vi "数据查询_仪器数据.vi"() -> ()   [LabVIEW 2016]
uses:
  <vilib>/Utility/miscctls.llb/LVRowAndColumnUnsignedTypeDef.ctl
  <vilib>/Utility/miscctls.llb/LVPointTypeDef.ctl
panel:
  in  "工作模式":string(combo)="全部数据"
  in  "查询":bool
  in  "结束日期":string="2020/01/01"
  in  "起始日期":string="2010/01/01"
  in  "组合框":string(combo)
  out "数据表":string[][](table)
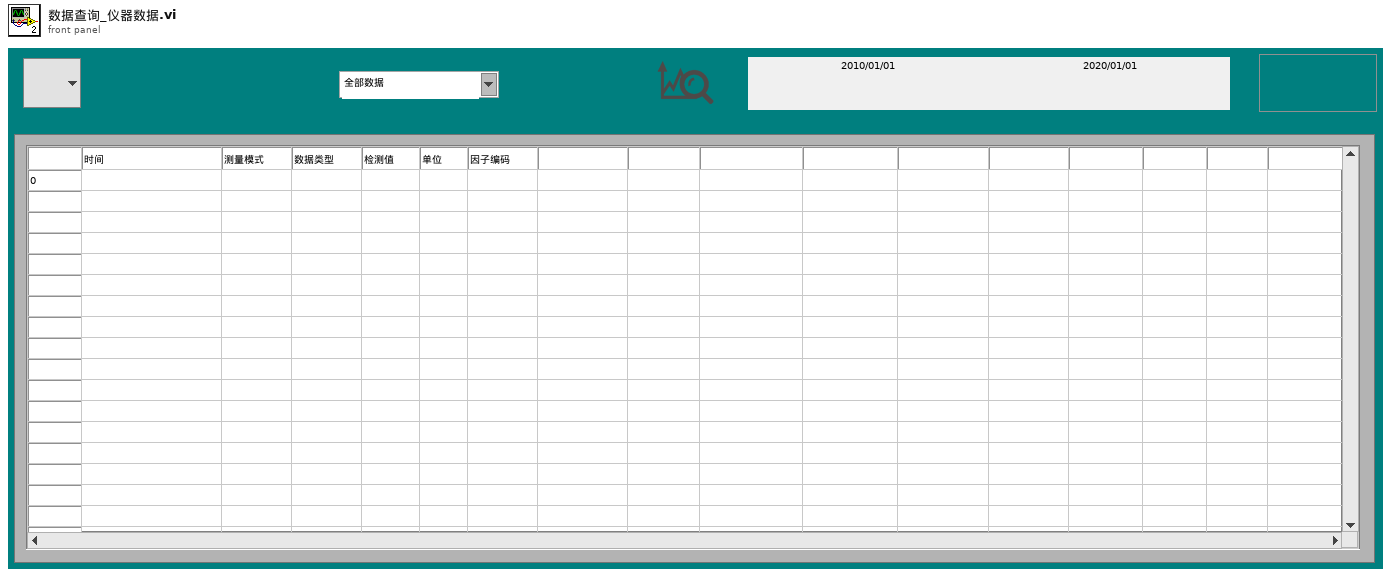
[diagram p1: front panel]
types:
  T1 = typedef "LVRowAndColumnUnsignedTypeDef.ctl" = cluster{"Row":u32, "Column":u32}
  T2 = typedef "LVPointTypeDef.ctl" = cluster{"Horizontal":i16, "Vertical":i16}
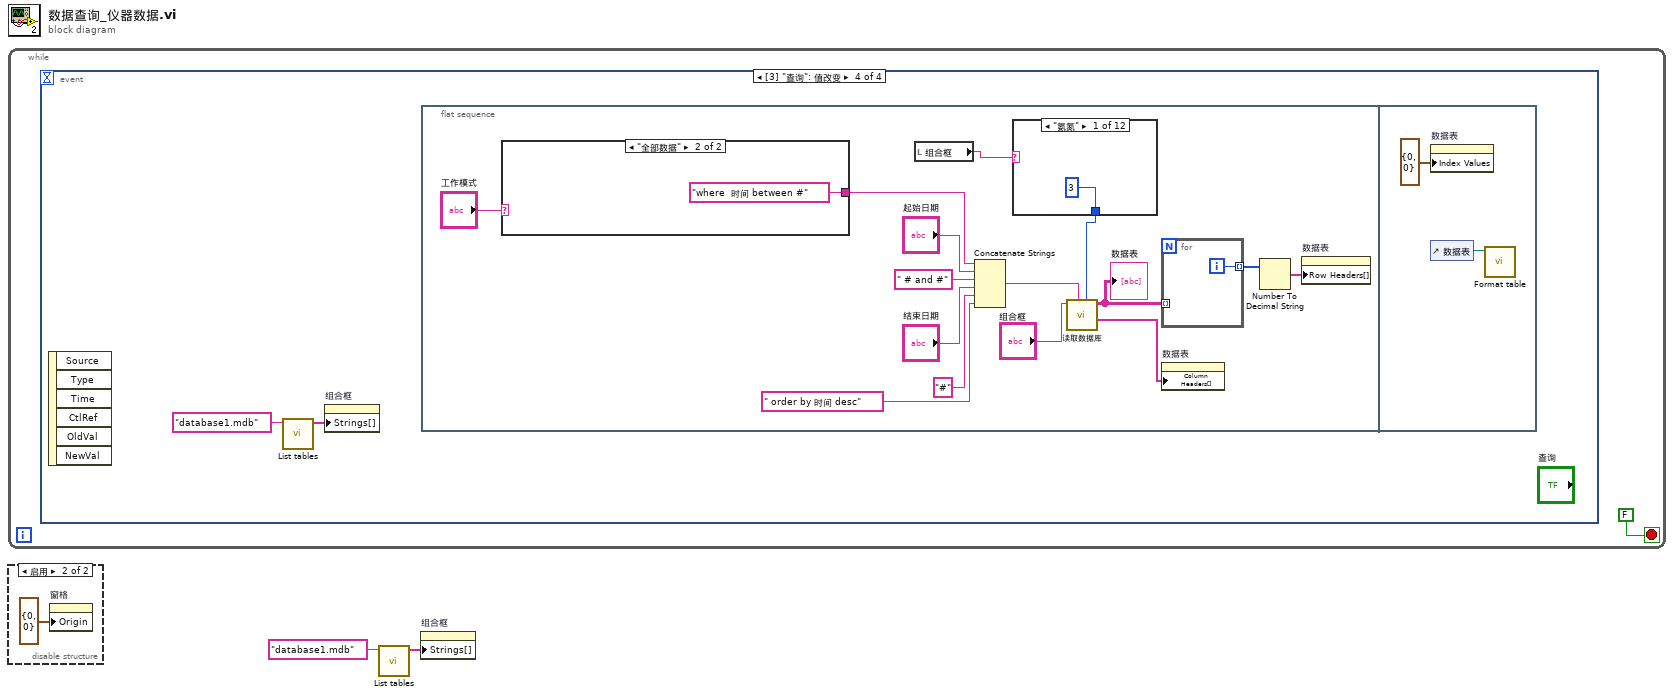
[diagram p0: block diagram]
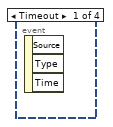
[diagram p2: hidden frame]
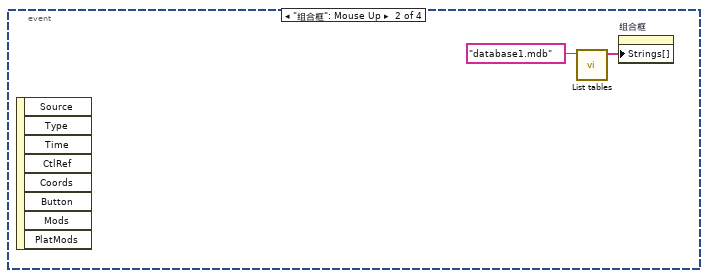
[diagram p3: hidden frame]
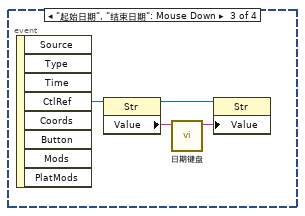
[diagram p4: hidden frame]
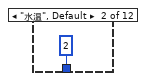
[diagram p5: hidden frame]
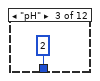
[diagram p6: hidden frame]
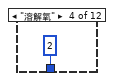
[diagram p7: hidden frame]
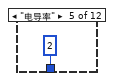
[diagram p8: hidden frame]
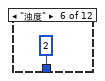
[diagram p9: hidden frame]
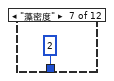
[diagram p10: hidden frame]
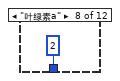
[diagram p11: hidden frame]
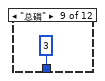
[diagram p12: hidden frame]
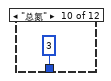
[diagram p13: hidden frame]
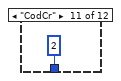
[diagram p14: hidden frame]
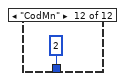
[diagram p15: hidden frame]
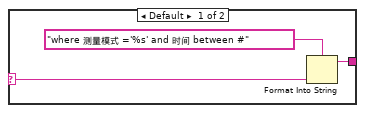
[diagram p16: hidden frame]
diagram:
  n1 = while {
    stop <- FALSE stop-if-true
    n2 = event shown="[3] \"查询\": 值改变" {
      selector: _ -> [_ _ _ _]
      dyn-events: _ -> [_ _ _ _]
      timeout: _ -> [_ _ _ _]
      event Timeout {
        n3 = event-data() -> ()  [unwired: 1 in, 3 out]
      }
      event "组合框": Mouse Up {
        n4 = event-data() -> ()  [unwired: 1 in, 8 out]
        n5 = call "List tables.vi"("database"="database1.mdb") -> ("tables"=w5:string[])  [unwired: 9 in, 1 out]
        n6 = property on="组合框" class="CmbBox"("Strings[]"=w5) -> ()  [unwired: 2 in, 2 out]
      }
      event "起始日期", "结束日期": Mouse Down {
        n7 = event-data() -> ("CtlRef"=w9:refnum<vi>)  [unwired: 1 in, 7 out]
        n8 = property class="Str"(reference=w9) -> (reference out=w7:refnum<vi>, "Value"=w8:string)  [unwired: 1 in, 1 out]
        n9 = call "日期键盘.vi"("原值"=w8) -> ("x+y"=w6:string)  [unwired: 10 in]
        n10 = property class="Str"(reference=w7, "Value"=w6) -> ()  [unwired: 1 in, 2 out]
      }
      event "查询": Value Change {
        n11 = event-data() -> ()  [unwired: 1 in, 6 out]
        n12 = call "List tables.vi"("database"="database1.mdb") -> ("tables"=w11:string[])  [unwired: 9 in, 1 out]
        n13 = property on="组合框" class="CmbBox"("Strings[]"=w11) -> ()  [unwired: 2 in, 2 out]
        n14 = flat-sequence {
          frame #0 {
            n15 = case shown="\"全部数据\"" "工作模式" {
              selector: "工作模式" -> [w41 _]
              tunnel: [w39 "where  时间 between #" ("condition")] -> w14
              frame Default {
                n16 = Format Into String(format string="where 测量模式 ='%s' and 时间 between #" ("condition"), w41) -> (resulting string=w39:string)  [unwired: 2 in, 1 out]
              }
              frame "全部数据" {
              }
            }
            n17 = local read "组合框"() -> (w13:string)
            n18 = Concatenate Strings(w14, "起始日期", " # and #" ("condition"), "结束日期", "#" ("condition"), " order by 时间 desc" ("字符串")) -> (w25:string)
            n19 = case shown="\"氨氮\"" w13 {
              tunnel: [i16 3 ("精度(6)") i16 2 ("精度(6)") i16 2 ("精度(6)") i16 2 ("精度(6)") i16 2 ("精度(6)") i16 2 ("精度(6)") i16 2 ("精度(6)") i16 2 ("精度(6)") i16 3 ("精度(6)") i16 3 ("精度(6)") i16 2 ("精度(6)") i16 2 ("精度(6)")] -> w12
              frame "氨氮" {
              }
              frame "水温", Default {
              }
              frame "pH" {
              }
              frame "溶解氧" {
              }
              frame "电导率" {
              }
              frame "浊度" {
              }
              frame "藻密度" {
              }
              frame "叶绿素a" {
              }
              frame "总磷" {
              }
              frame "总氮" {
              }
              frame "CodCr" {
              }
              frame "CodMn" {
              }
            }
            n20 = call "读取数据库.vi"("精度(6)"=w12, "condition"=w25, "组合框"="组合框") -> ("columns"=w21:string[], "表格"=w18:string[][])  [unwired: 5 in, 2 out]
            "数据表" <- w18
            n21 = for {
              tunnel: w18 -> [_] mode=indexing
              tunnel: [w43] -> w17 mode=indexing
              i -> [w43]
            }
            n22 = property on="数据表" class="Tbl (严格)"("Column Headers[]"=w21) -> ()  [unwired: 2 in, 2 out]
            n23 = Number To Decimal String(number=w17) -> (decimal integer string=w16:string[])  [unwired: 1 in]
            n24 = property on="数据表" class="Tbl (严格)"("Row Headers[]"=w16) -> ()  [unwired: 2 in, 2 out]
          }
          frame #1 {
            n25 = property on="数据表" class="Tbl (严格)"("Index Values"=T1 {"Row"=0, "Column"=0} ("索引值")) -> ()  [unwired: 2 in, 2 out]
            n26 = control-ref of="数据表"() -> (w44:refnum<vi>)
            n27 = call "Format table.vi"("Table输入"=w44) -> ()  [unwired: 11 in]
          }
        }
      }
    }
  }
  n28 = disable-structure shown="启用" {
    frame Disabled {
    }
    frame Enabled {
      n29 = property on="窗格" class="Pane"("Origin"=T2 {"Horizontal"=0, "Vertical"=0} ("原点")) -> ()  [unwired: 2 in, 2 out]
    }
  }
  n30 = call "List tables.vi"("database"="database1.mdb") -> ("tables"=w1:string[])  [unwired: 9 in, 1 out]
  n31 = property on="组合框" class="CmbBox"("Strings[]"=w1) -> ()  [unwired: 2 in, 2 out]
